vi "subEstimateChannel.vi"(0 "Data Stream In":cdb[][](array[numeric]), 1 "bits/symbol":i32, 9 "System Parameters":T1={"Symbol Rate"=64.0, "Symbols per Packet"=8, "Tx Oversample Factor"=16, "Rx Oversample Factor"=16, "Modulation Scheme"=enum."4-QAM", "filter length (symbols)"=8, "filter parameter"=0.5, "Training Sequence"=[], "Channel Length Estimate"=4, "Frequency Offset\nCorrection?"=TRUE} {"Symbol Rate" format="%#_6p"; "Training Sequence" format="%#_3p"; "filter parameter" format="%.2f"}, 11 "error in (no error)":errorcluster) -> (4 "Symbols Out":cdb[][](array[numeric]), 6 "h[n]":cdb[][][](array[numeric]), 15 "error out":errorcluster)   [LabVIEW 2011]
uses:
  ModulationParameters.ctl
panel:
  out "mean squared errors":dbl[][](array[numeric])
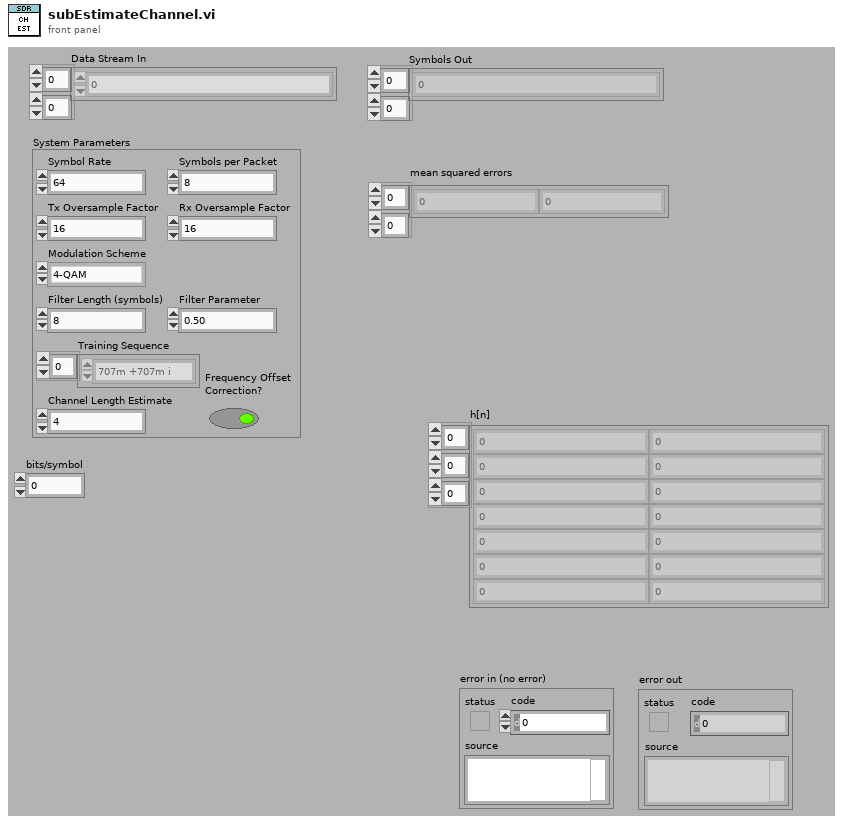
[diagram p1: front panel]
types:
  T1 = typedef "ModulationParameters.ctl" = cluster{"Symbol Rate":dbl, "Symbols per Packet":i32, "Tx Oversample Factor":i32, "Rx Oversample Factor":i32, "Modulation Scheme":enum16{"4-QAM", "16-QAM", "64-QAM"}, "filter length (symbols)":i32, "filter parameter":dbl, "Training Sequence":cdb[], "Channel Length Estimate":i32, "Frequency Offset\nCorrection?":bool}
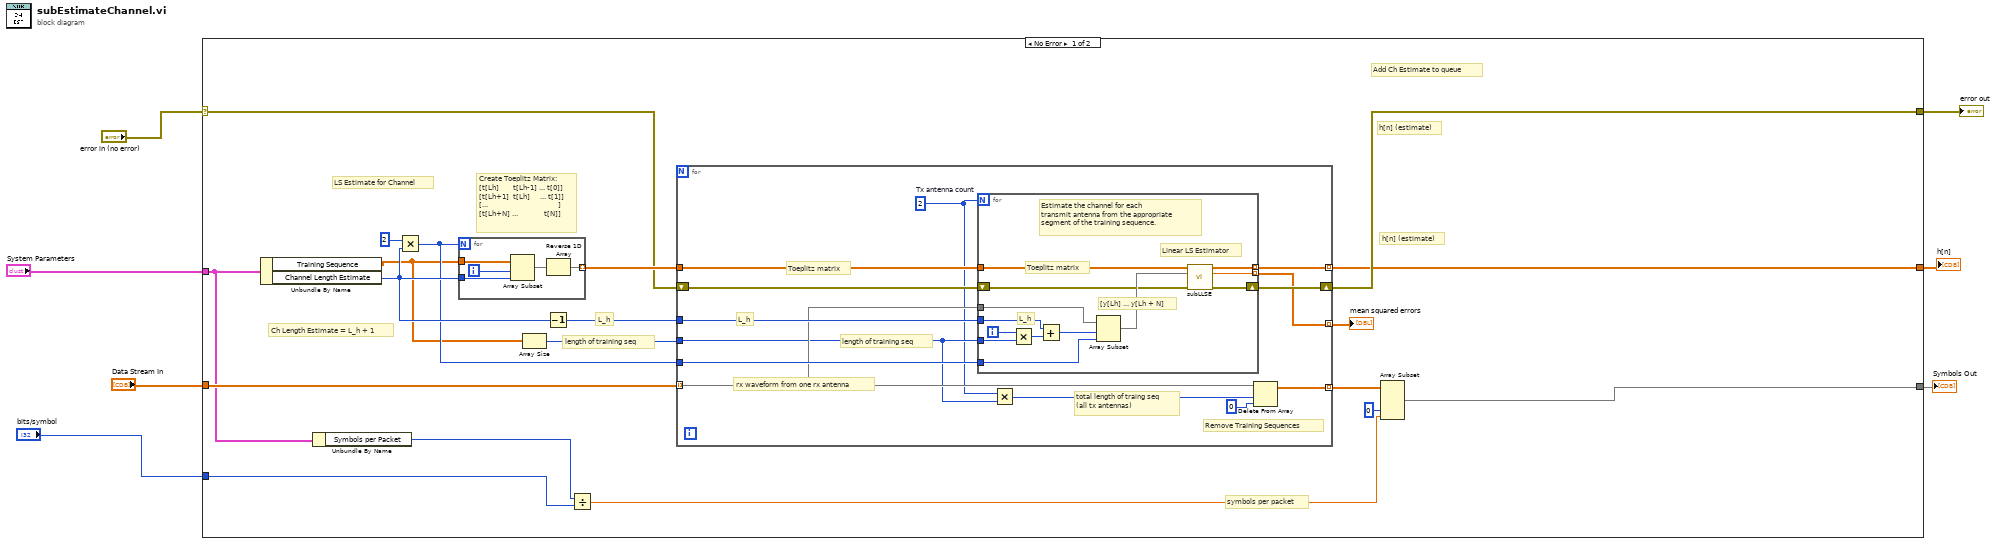
[diagram p0: block diagram]
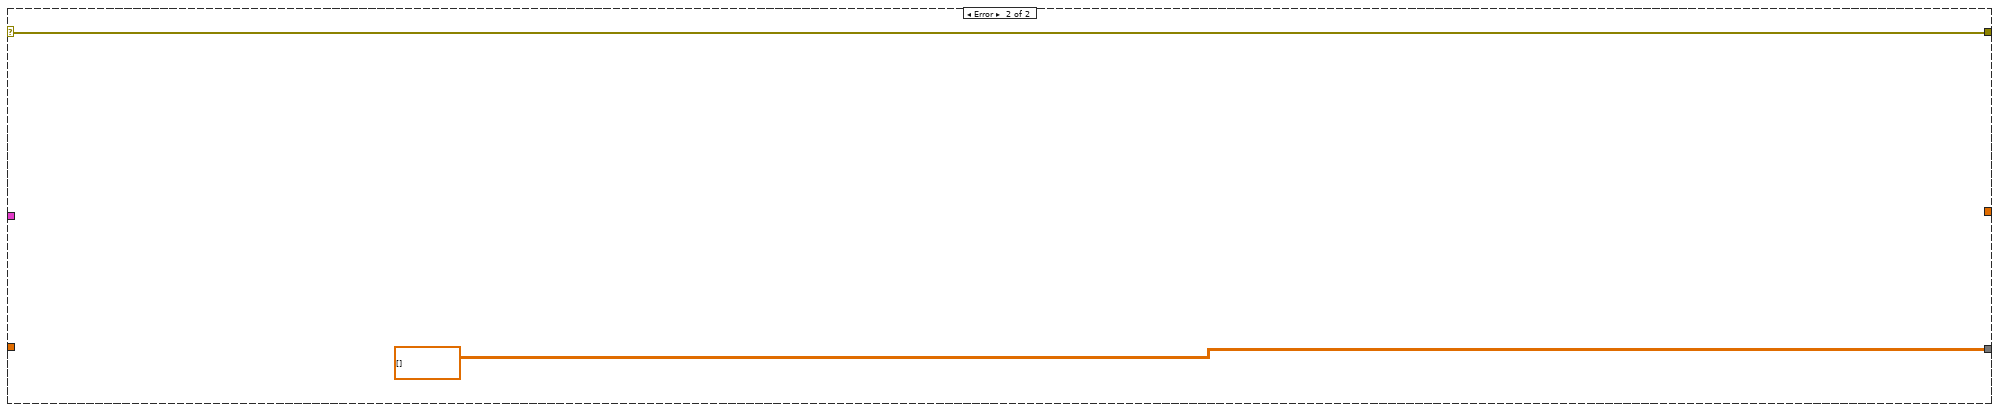
[diagram p2: hidden frame]
diagram:
  n1 = case shown="No Error" "error in (no error)" {
    selector: "error in (no error)" -> [w19 w59]
    tunnel: [w11 w59] -> w6
    tunnel: "Data Stream In" -> [w12 _]
    tunnel: "System Parameters" -> [w9 _]
    tunnel: [w13 cdb[][] []] -> w3
    tunnel: [w10 _] -> w2
    tunnel: "bits/symbol" -> [w8 _]
    frame No Error {
      # "symbols per packet"
      # "h[n] (estimate)"
      # "L_h"
      # "length of training seq"
      # "h[n] (estimate)"
      # "Add Ch Estimate to queue"
      # "Ch Length Estimate = L_h + 1"
      # "Create Toeplitz Matrix:\n[t[Lh]       t[Lh-1] ... t[0]]\n[t[Lh+1]  t[Lh]     ... t[1]]\n[...                                   ]\n[t[Lh+N] ...             t[N]]"
      # "LS Estimate for Channel"
      n2 = Unbundle By Name(w9) -> ("Training Sequence"=w21:cdb[], "Channel Length Estimate"=w25:i32)
      n3 = Unbundle By Name(w9) -> ("Symbols per Packet"=w15:i32)
      n4 = Multiply(x=2, y=w25) -> (x*y=w23:i32)
      n5 = for {
        N: w23 -> [_]
        tunnel: w21 -> [w57]
        tunnel: w25 -> [w55]
        tunnel: [w53] -> w22 mode=indexing
        i -> [w56]
        n6 = Array Subset(array=w57, index=w56, length=w55) -> (w54:cdb[])
        n7 = Reverse 1D Array(array=w54) -> (reversed array=w53:cdb[])
      }
      n8 = Array Size(array=w21) -> (size(s)=w20:i32)
      n9 = Decrement(x=w25) -> (x-1=w24:i32)
      n10 = Divide(x=w15, y=w8) -> (x/y=w14:dbl)
      n11 = for {
        tunnel: w24 -> [w39]
        tunnel: w23 -> [w38]
        tunnel: w22 -> [w37]
        tunnel: w20 -> [w31]
        tunnel: w12 -> [w32] mode=indexing
        tunnel: [w33] -> w17 mode=indexing
        shift-right: [w35] -> w11
        shift-left: w19 -> [w36]
        tunnel: [w29] -> w10 mode=indexing
        tunnel: [w28] -> w18 mode=indexing
        w27 = 2  # Tx antenna count
        # "Remove Training Sequences"
        # "L_h"
        # "Toeplitz matrix"
        # "rx waveform from one rx antenna"
        # "total length of traing seq\n(all tx antennas)"
        # "length of training seq"
        n12 = for {
          N: w27 -> [_]
          tunnel: w39 -> [w44]
          tunnel: w38 -> [w52]
          tunnel: w37 -> [w50]
          tunnel: w32 -> [w47]
          tunnel: w31 -> [w45]
          shift-right: [w48] -> w35
          shift-left: w36 -> [w49]
          tunnel: [w41] -> w29 mode=indexing
          tunnel: [w40] -> w28 mode=indexing
          i -> [w46]
          # "L_h"
          # "Estimate the channel for each\ntransmit antenna from the appropriate\nsegment of the training sequence."
          # "Toeplitz matrix"
          # "Linear LS Estimator"
          # "[y[Lh] ... y[Lh + N]"
          n13 = Multiply(x=w46, y=w45) -> (x*y=w43:i32)
          n14 = Add(x=w44, y=w43) -> (x+y=w42:i32)
          n15 = Array Subset(array=w47, index=w42, length=w52) -> (w51:cdb[])
          n16 = call "subLLSE.vi"("A"=w50, "b"=w51, "error in (no error)"=w49) -> ("x.estimate"=w41:cdb[], "mean square error"=w40:dbl, "error out"=w48:errorcluster)  [unwired: 10 in]
        }
        n17 = Multiply(x=w27, y=w31) -> (x*y=w30:i32)
        n18 = Delete From Array(array=w32, length=w30, index=0) -> (array with subset deleted=w33:cdb[])  [unwired: 1 out]
      }
      "mean squared errors" <- w18
      n19 = Array Subset(array=w17, index (col)=0 ("index"), length (col)=w14) -> (w13:cdb[][])  [unwired: 2 in]
    }
    frame Error {
    }
  }
  "error out" <- w6
  "Symbols Out" <- w3
  "h[n]" <- w2
